vi "Turret Motion.vi"   [LabVIEW 2011]
uses:
  Robot Global Data.vi
  <vilib>/addons/control/pid/pid.llb/PID (DBL).vi
  <vilib>/addons/control/pid/NI_PID_pid.lvlib
types:
  T1 = cluster{"proportional gain (Kc)":dbl, "integral time (Ti, min)":dbl, "derivative time (Td, min)":dbl}
  T2 = typedef "WPI_MotorControlDeviceRef.ctl" = cluster{"DeviceStatus":errorcluster, "Type":enum16{"PWM", "CAN"}, "PWM":cluster{"Digital Module":T3, "PWM Channel":T4, "DeadBand":T5}, "CAN":cluster{"Device Number":u8, "Control Mode":T6, "Semaphore":T7, "Max Vout":dbl}, "Invert":bool, "TransformRef":T8, "InvTransformRef":T8}
  T3 = typedef "FPGA_TypedefDigitalModule.ctl" = enum16{"Digital Module 1", "Digital Module 2"}
  T4 = typedef "FPGA_DIOPWMChannel.ctl" = enum8{"PWM 1", "PWM 2", "PWM 3", "PWM 4", "PWM 5", "PWM 6", "PWM 7", "PWM 8", "PWM 9", "PWM 10", "Invalid"}
  T5 = typedef "WPI_PWMDeadband.ctl" = cluster{"Name":string, "maxPositivePwm":i32, "minPositivePwm":i32, "centerPwm":i32, "maxNegativePwm":i32, "minNegativePwm":i32, "angularRange":u16}
  T6 = typedef "WPI_CANJaguar_ControlMode.ctl" = enum8{"Percent VBus", "Current", "Speed", "Position", "Voltage"}
  T7 = typedef "Semaphore RefNum" = refnum<k1>
  T8 = typedef "WPI_PWMTransform_ConPane.ctl" = refnum<vi>
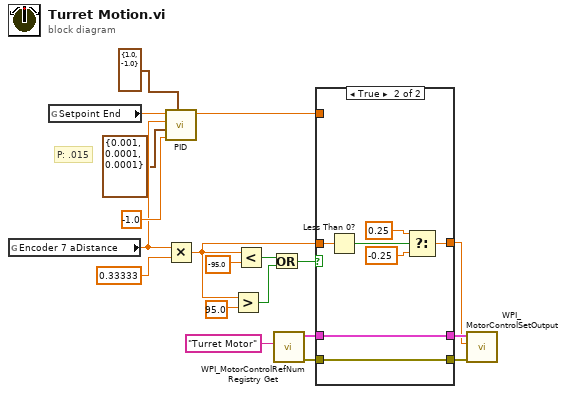
[diagram p0: block diagram]
diagram:
  # "P: .015"
  n1 = global read "Robot Global Data.vi" "Encoder 7 aDistance"() -> (w4:dbl)
  n2 = global read "Robot Global Data.vi" "Setpoint End"() -> (w3:dbl)
  n3 = call-poly <vilib>:"PID.vi"("output range"=cluster{"output high":dbl, "output low":dbl} {"output high"=1.0, "output low"=-1.0}, "dt (s)"=-1.0, "PID gains"=T1 {"proportional gain (Kc)"=0.001, "integral time (Ti, min)"=0.0001, "derivative time (Td, min)"=0.0001}, "process variable"=w4, "setpoint"=w3) -> ("output"=w15:dbl)  [unwired: 5 in, 1 out]
  n4 = Multiply(x=w4, y=0.33333) -> (x*y=w7:dbl)
  n5 = Greater?(x=w7, y=95.0) -> (0:w8:bool)
  n6 = Less?(x=w7, y=-95.0) -> (x < y?=w9:bool)
  n7 = Or(x=w9, y=w8) -> (x .or. y?=w5:bool)
  n8 = call <vilib>:"WPI_MotorControlRefNum Registry Get.vi"("refnum name"="Turret Motor") -> ("error out"=w18:errorcluster, "MotorControlDevRef"=w17:T2)  [unwired: 9 in]
  n9 = case shown="True" w5 {
    tunnel: w18 -> [w20 w28]
    tunnel: w17 -> [w21 w29]
    tunnel: w15 -> [w22 _]
    tunnel: [w21 w29] -> w11
    tunnel: [w20 w28] -> w10
    tunnel: w7 -> [_ w27]
    tunnel: [w22 w23] -> w6
    frame False {
    }
    frame True {
      n10 = Less Than 0?(x=w27) -> (x < 0?=w26:bool)
      n11 = Select(t=0.25, s=w26, f=-0.25) -> (s? t:f=w23:dbl)
    }
  }
  n12 = call <vilib>:"WPI_MotorControlSetOutput.vi"("error in (no error)"=w10, "Output"=w6, "MotorControlDevRef"=w11) -> ()  [unwired: 7 in, 2 out]
